vi "Get Task Attribute Wrapper.vi"(0 "Task map in":map{string, refnum<k21>}(c390), 5 "Message Data in":T2, 11 "error in (no error)":errorcluster) -> (4 "Task map out":map{string, refnum<k21>}(c390), 6 "Message Data out":T1, 15 "error out":errorcluster)   [LabVIEW 2021, in "NI DAQmx_wrapper.lvlib"]
uses:
  NI DAQmx_wrapper.lvlib
  NI DAQmx_server/RPC Messages/nidaqmx_grpc_GetTaskAttributeStringRequest.ctl
  NI DAQmx_server/RPC Messages/nidevice_grpc_Session_session/nidevice_grpc_Session_session.lvclass
  NI DAQmx_server/RPC Messages/nidaqmx_grpc_GetTaskAttributeStringRequest_attribute_enum/nidaqmx_grpc_GetTaskAttributeStringRequest_attribute_enum.lvclass
  NI DAQmx_server/RPC Messages/nidevice_grpc_Session.ctl
  NI DAQmx_server/RPC Messages/nidaqmx_grpc_GetTaskAttributeStringResponse.ctl
  NI DAQmx_server/RPC Messages/nidaqmx_grpc_GetTaskAttributeStringRequest_attribute_enum/nidaqmx_grpc_GetTaskAttributeStringRequest_attribute_enum.lvclass/nidaqmx_grpc_GetTaskAttributeStringRequest_attribute_enum.ctl
  NI DAQmx_server/RPC Messages/nidevice_grpc_Session_session/nidevice_grpc_Session_session.lvclass/nidevice_grpc_Session_session.ctl
  <resource>/objmgr/daqmx.rc
  NI DAQmx_server/NI DAQmx_server.lvlib
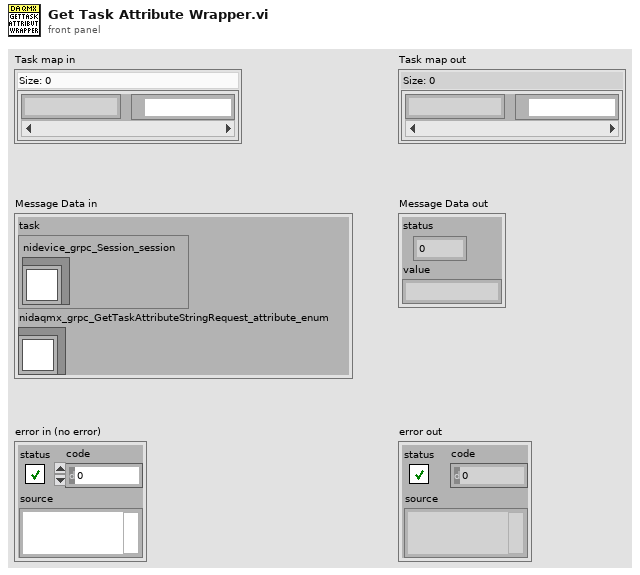
[diagram p1: front panel]
types:
  T1 = typedef "NI DAQmx_server.lvlib/nidaqmx_grpc_GetTaskAttributeStringResponse.ctl" = cluster{"status":i32, "value":string}
  T2 = typedef "NI DAQmx_server.lvlib/nidaqmx_grpc_GetTaskAttributeStringRequest.ctl" = cluster{"task":T3, "nidaqmx_grpc_GetTaskAttributeStringRequest_attribute_enum":refnum<class "nidaqmx_grpc_GetTaskAttributeStringRequest_attribute_enum.lvclass">}
  T3 = typedef "NI DAQmx_server.lvlib/nidevice_grpc_Session.ctl" = cluster{"nidevice_grpc_Session_session":refnum<class "nidevice_grpc_Session_session.lvclass">}
  T4 = typedef "NI DAQmx_server.lvlib/nidaqmx_grpc_TaskStringAttribute.ctl" = enum32{"TASK_STRING_ATTRIBUTE_UNSPECIFIED", "TASK_ATTRIBUTE_CHANNELS", "TASK_ATTRIBUTE_NAME", "TASK_ATTRIBUTE_DEVICES"}
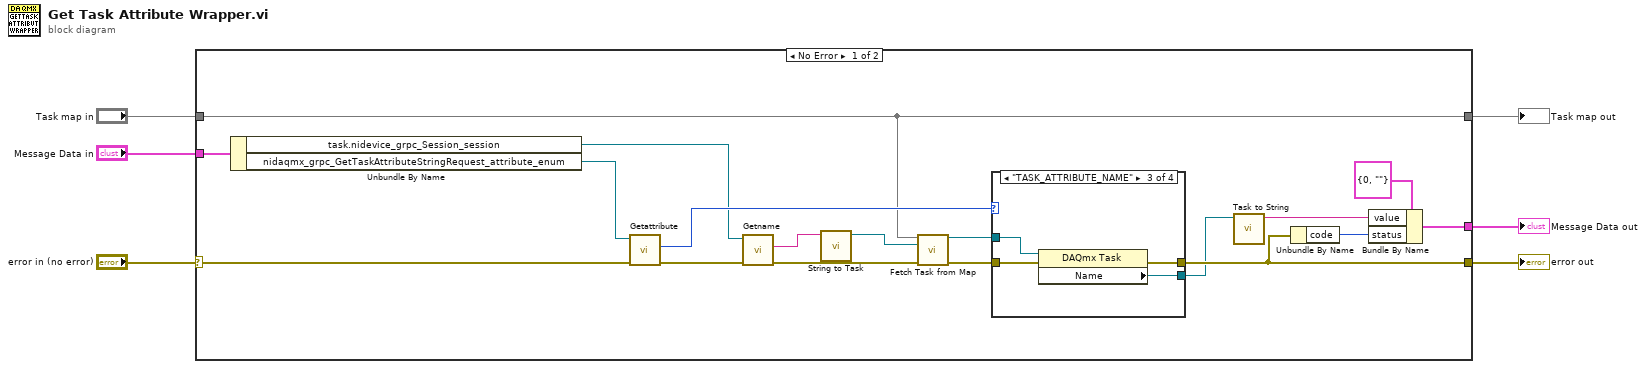
[diagram p0: block diagram]
diagram:
  n1 = case shown="No Error" "error in (no error)" {
    selector: "error in (no error)" -> [w23 w33]
    tunnel: [w11 w33] -> w5
    tunnel: "Task map in" -> [w15 w32]
    tunnel: [w15 w32] -> w3
    tunnel: "Message Data in" -> [w24 _]
    tunnel: [w7 _] -> w1
    frame No Error {
      n2 = Unbundle By Name(w24) -> ("task.nidevice_grpc_Session_session"=w16:refnum<class "nidevice_grpc_Session_session.lvclass">, "nidaqmx_grpc_GetTaskAttributeStringRequest_attribute_enum"=w22:refnum<class "nidaqmx_grpc_GetTaskAttributeStringRequest_attribute_enum.lvclass">)
      n3 = call "Getattribute.vi"("error in (no error)"=w23, "OneOfTemplate in"=w22) -> ("error out"=w18:errorcluster, "Get_Val"=w17:T4)  [unwired: 7 in, 1 out]
      n4 = call "Getname.vi"("error in (no error)"=w18, "OneOfTemplate in"=w16) -> ("error out"=w19:errorcluster, "Get_Val"=w21:string)  [unwired: 7 in, 1 out]
      n5 = call "String to Task.vi"("Get_Val"=w21) -> ("Refnum out"=w20:refnum<k21>)  [unwired: 10 in]
      n6 = call "Fetch Task from Map.vi"("Task map in"=w15, "Task in"=w20, "error in (no error)"=w19) -> ("Task out"=w13:refnum<k21>, "error out"=w14:errorcluster)  [unwired: 10 in, 1 out]
      n7 = case shown="\"TASK_ATTRIBUTE_NAME\"" w17 {
        tunnel: w14 -> [w25 w26 w30 w31]
        tunnel: w13 -> [_ _ w28 _]
        tunnel: [w25 w26 w29 w31] -> w11
        tunnel: [_ _ w27 _] -> w8
        frame "TASK_STRING_ATTRIBUTE_UNSPECIFIED", Default {
        }
        frame "TASK_ATTRIBUTE_CHANNELS" {
        }
        frame "TASK_ATTRIBUTE_NAME" {
          n8 = property class="DAQmx Task"(reference=w28, error in=w30) -> (error out=w29:errorcluster, "Name"=w27:refnum<k21>)  [unwired: 1 out]
        }
        frame "TASK_ATTRIBUTE_DEVICES" {
        }
      }
      n9 = call "Task to String.vi"("Refnum in"=w8) -> ("String"=w9:string)  [unwired: 10 in]
      n10 = Unbundle By Name(w11) -> ("code"=w12:i32)
      n11 = Bundle By Name(cluster=T1 {"status"=0, "value"=""} ("Message Data 2"), "value"=w9, "status"=w12) -> (w7:T1)
    }
    frame Error {
    }
  }
  "error out" <- w5
  "Task map out" <- w3
  "Message Data out" <- w1
